vi "Configure Trigger (Runt).vi"(0 "VISA resource name":refnum<visa-resource-name>, 1 "Trigger Polarity (0: Positive)":u16(ring) items=["Positive", "Negative", "Either"], 5 "Trigger Source (0: Channel 1)":u16(ring) items=["Channel 1", "Channel 2", "Channel 3", "Channel 4", "RF"], 7 "High Threshold (0.8V)":dbl=0.8, 9 "Low Threshold (0.0V)":dbl, 11 "error in (no error)":errorcluster, 12 "Trigger Condition (0: Occurs)":u16(ring) items=["Occurs", "Less Than", "More Than", "Equal", "Not Equal"], 13 "Runt Width (4.0ns)":dbl=4e-09) -> (4 "VISA resource name out":refnum<visa-resource-name>, 15 "error out":errorcluster)   [LabVIEW 2013, in "Tektronix DPO MSO 2000 4000 Series.lvlib"]
doc: "Configures runt trigger settings for an oscilloscope. A runt trigger occurs when the trigger signal crosses one of the runt thresholds twice without crossing the other runt threshold."
uses:
  Tektronix DPO MSO 2000 4000 Series.lvlib
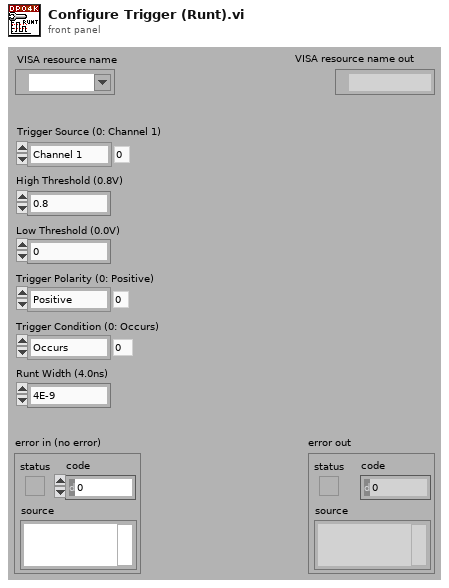
[diagram p1: front panel]
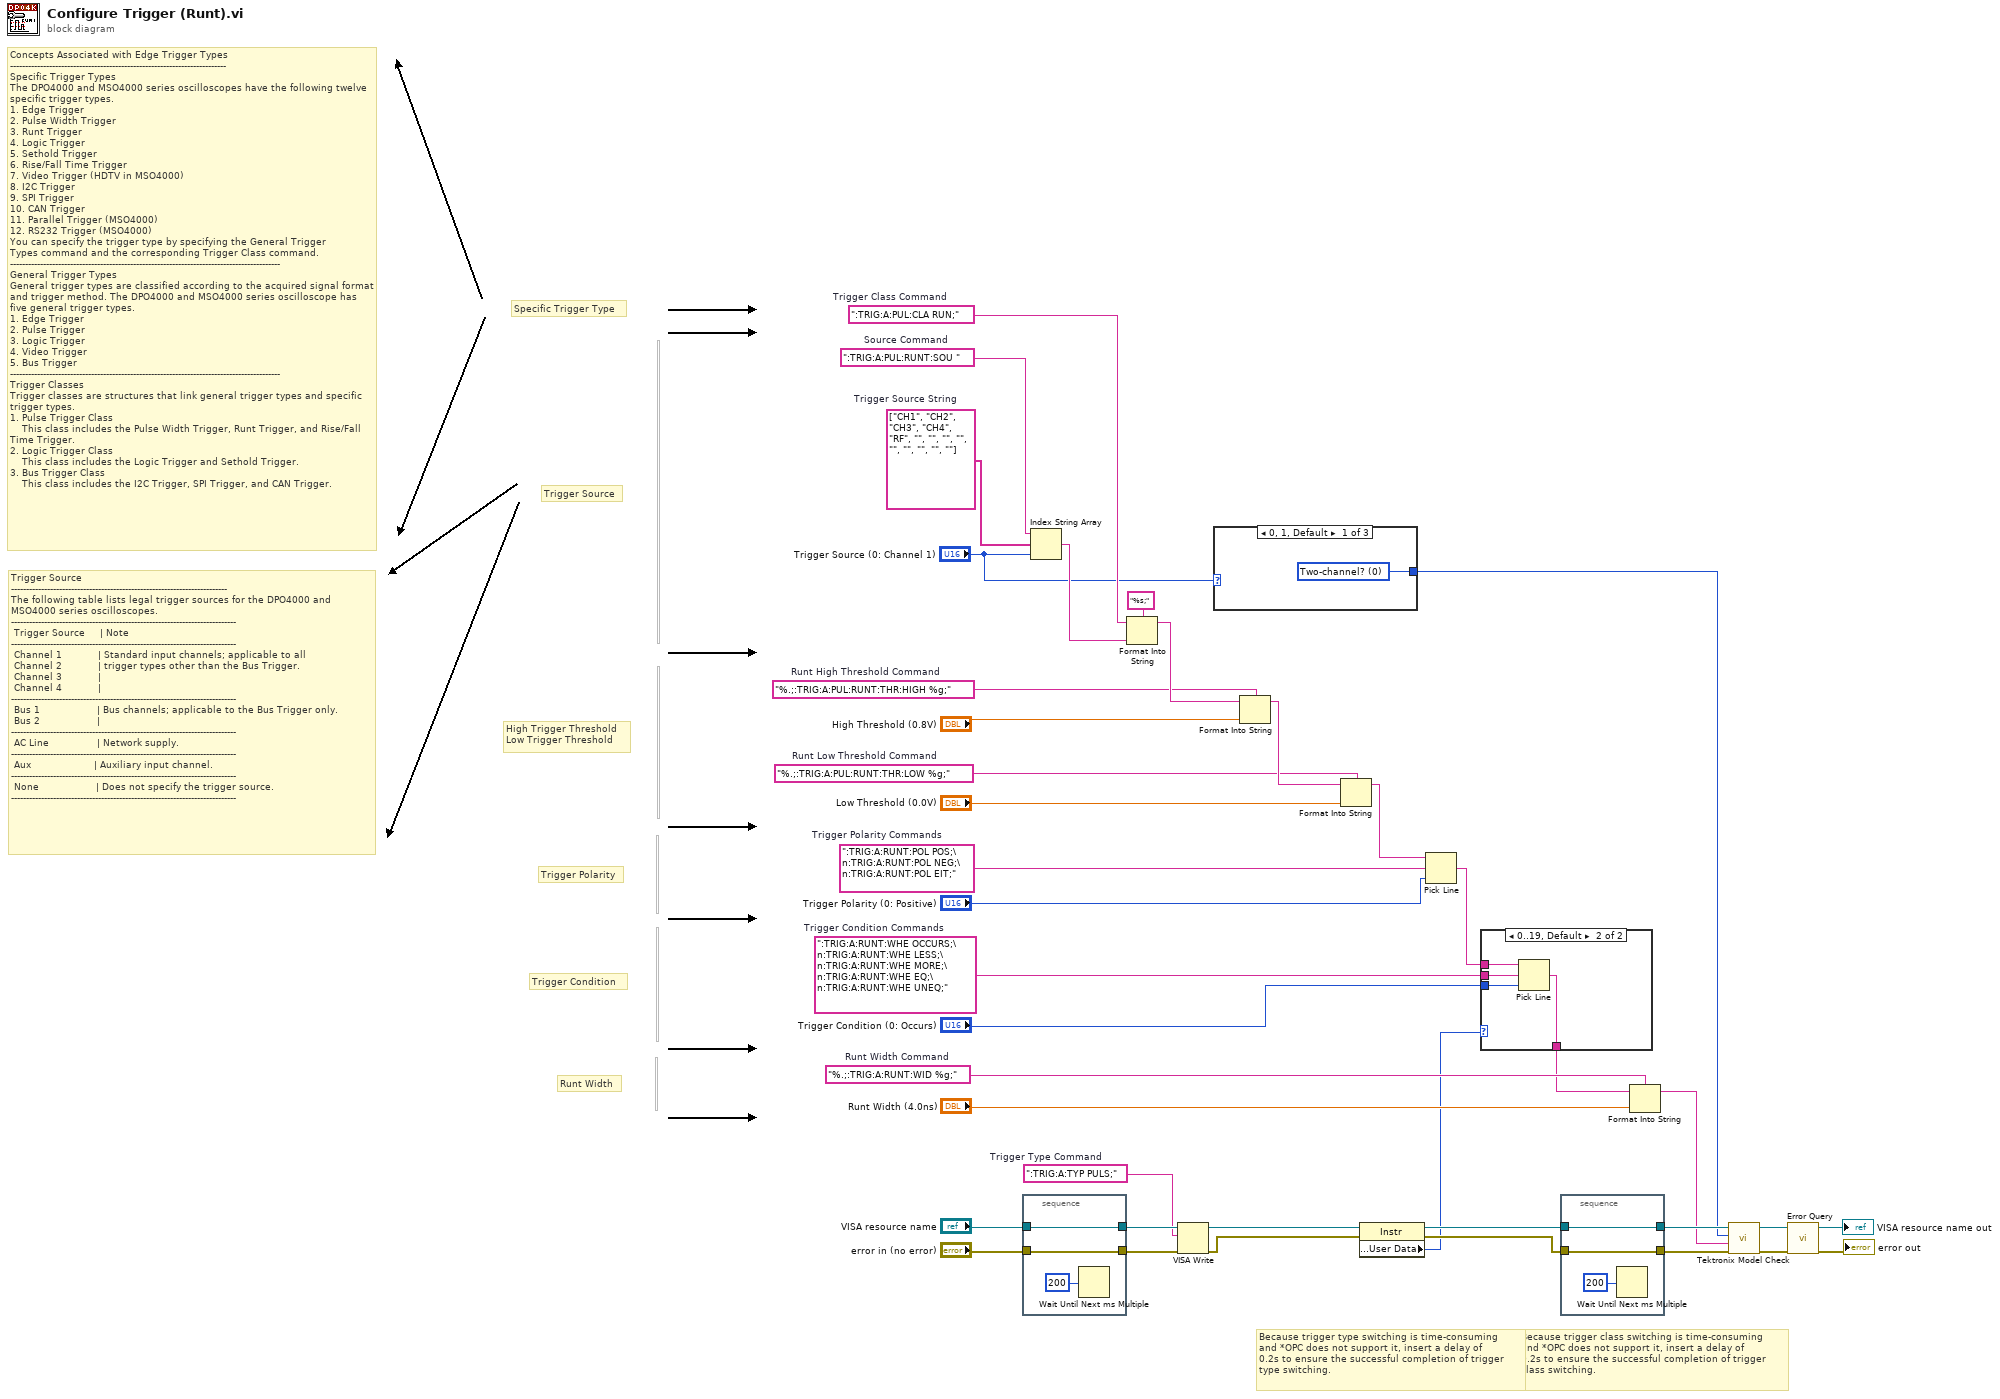
[diagram p0: block diagram]
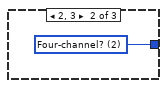
[diagram p2: hidden frame]
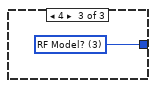
[diagram p3: hidden frame]
diagram:
  w17 = string[] ["CH1", "CH2", "CH3", "CH4", "RF", "", "", "", "", "", "", "", "", ""]  # Trigger Source String
  w21 = "%.;:TRIG:A:RUNT:WID %g;"  # Runt Width Command
  w24 = ":TRIG:A:RUNT:WHE OCCURS;\n:TRIG:A:RUNT:WHE LESS;\n:TRIG:A:RUNT:WHE MORE;\n:TRIG:A:RUNT:WHE EQ;\n:TRIG:A:RUNT:WHE UNEQ;"  # Trigger Condition Commands
  w26 = ":TRIG:A:RUNT:POL POS;\n:TRIG:A:RUNT:POL NEG;\n:TRIG:A:RUNT:POL EIT;"  # Trigger Polarity Commands
  w28 = "%.;:TRIG:A:PUL:RUNT:THR:LOW %g;"  # Runt Low Threshold Command
  w30 = "%.;:TRIG:A:PUL:RUNT:THR:HIGH %g;"  # Runt High Threshold Command
  w36 = ":TRIG:A:PUL:RUNT:SOU "  # Source Command
  w34 = ":TRIG:A:PUL:CLA RUN;"  # Trigger Class Command
  w37 = ":TRIG:A:TYP PULS;"  # Trigger Type Command
  # "Trigger Source\n------------------------------------------------------------------------\nThe following table lists legal trigger sources for the DPO4000 and MSO4000 series oscilloscopes.\n---------------------------------------------------------------------------\n Trigger Source     | Note                                                           \n---------------------------------------------------------------------------\n Channel 1            | Standard input channels; applicable to all      \n Channel 2            | trigger types other than the Bus Trigger.         \n Channel 3            |     \n Channel 4            |\n---------------------------------------------------------------------------\n Bus 1                   | Bus channels; applicable to the Bus Trigger only.\n Bus 2                   | \n---------------------------------------------------------------------------\n AC Line                | Network supply.\n---------------------------------------------------------------------------\n Aux                     | Auxiliary input channel.\n---------------------------------------------------------------------------\n None                   | Does not specify the trigger source.\n---------------------------------------------------------------------------"
  # "Concepts Associated with Edge Trigger Types\n------------------------------------------------------------------------\nSpecific Trigger Types\nThe DPO4000 and MSO4000 series oscilloscopes have the following twelve specific trigger types.\n1. Edge Trigger\n2. Pulse Width Trigger\n3. Runt Trigger\n4. Logic Trigger\n5. Sethold Trigger\n6. Rise/Fall Time Trigger\n7. Video Trigger (HDTV in MSO4000)\n8. I2C Trigger\n9. SPI Trigger\n10. CAN Trigger\n11. Parallel Trigger (MSO4000)\n12. RS232 Trigger (MSO4000)\nYou can specify the trigger type by specifying the General Trigger \nTypes command and the corresponding Trigger Class command.\n------------------------------------------------------------------------------------------\nGeneral Trigger Types \nGeneral trigger types are classified according to the acquired signal format and trigger method. The DPO4000 and MSO4000 series oscilloscope has five general trigger types.\n1. Edge Trigger\n2. Pulse Trigger\n3. Logic Trigger\n4. Video Trigger\n5. Bus Trigger\n------------------------------------------------------------------------------------------\nTrigger Classes\nTrigger classes are structures that link general trigger types and specific trigger types.\n1. Pulse Trigger Class\n    This class includes the Pulse Width Trigger, Runt Trigger, and Rise/Fall Time Trigger.\n2. Logic Trigger Class\n    This class includes the Logic Trigger and Sethold Trigger.\n3. Bus Trigger Class\n    This class includes the I2C Trigger, SPI Trigger, and CAN Trigger."
  # "Because trigger class switching is time-consuming\nand *OPC does not support it, insert a delay of\n0.2s to ensure the successful completion of trigger\nclass switching."
  # "Because trigger type switching is time-consuming\nand *OPC does not support it, insert a delay of\n0.2s to ensure the successful completion of trigger\ntype switching."
  # "Runt Width"
  # "Trigger Condition"
  # "Trigger Polarity"
  # "High Trigger Threshold\nLow Trigger Threshold"
  # "Trigger Source"
  # "Specific Trigger Type"
  n1 = stacked-sequence {
    tunnel: "VISA resource name" -> [w41]
    tunnel: [w41] -> w39
    tunnel: "error in (no error)" -> [w40]
    tunnel: [w40] -> w38
    frame #0 {
      n2 = Wait Until Next ms Multiple(millisecond multiple=u32 200) -> ()  [unwired: 1 out]
    }
  }
  n3 = Index String Array(1:"Trigger Source (0: Channel 1)", 2:w17, 3:w36) -> (0:w35:string)
  n4 = Format Into String(format string="%s;", initial string=w34, w35) -> (resulting string=w32:string)  [unwired: 1 in, 1 out]
  n5 = VISA Write(VISA resource name=w39, write buffer=w37, error in (no error)=w38) -> (VISA resource name out=w12:refnum<visa-resource-name>, error out=w11:errorcluster)  [unwired: 1 out]
  n6 = case shown="0, 1, Default" "Trigger Source (0: Channel 1)" {
    tunnel: [w43 w44 w45] -> w1
    frame 0, 1, Default {
      w43 = u16 0 items=["Two-channel?", "Digital Model?", "Four-channel?", "RF Model?"] ("Oscilloscope Model Tests (3: RF Model?)")
    }
    frame 2, 3 {
      w44 = u16 2 items=["Two-channel?", "Digital Model?", "Four-channel?", "RF Model?"] ("Oscilloscope Model Tests (3: RF Model?)")
    }
    frame 4 {
      w45 = u16 3 items=["Two-channel?", "Digital Model?", "Four-channel?", "RF Model?"] ("Oscilloscope Model Tests (3: RF Model?)")
    }
  }
  n7 = Format Into String(format string=w30, initial string=w32, "High Threshold (0.8V)") -> (resulting string=w29:string)  [unwired: 1 in, 1 out]
  n8 = Format Into String(format string=w28, initial string=w29, "Low Threshold (0.0V)") -> (resulting string=w16:string)  [unwired: 1 in, 1 out]
  n9 = property class="Instr"(reference=w12, error in=w11) -> (reference out=w10:refnum<visa-resource-name>, error out=w9:errorcluster, "General Settings:User Data"=w8:u32)
  n10 = Pick Line(string ("")=w16, multi-line string=w26, line index="Trigger Polarity (0: Positive)") -> (output string=w15:string)
  n11 = case shown="0..19, Default" w8 {
    tunnel: w24 -> [_ w50]
    tunnel: "Trigger Condition (0: Occurs)" -> [_ w49]
    tunnel: [w46 w48] -> w20
    tunnel: w15 -> [w46 w47]
    frame 20, 27 {
    }
    frame 0..19, Default {
      n12 = Pick Line(string ("")=w47, multi-line string=w50, line index=w49) -> (output string=w48:string)
    }
  }
  n13 = stacked-sequence {
    tunnel: w10 -> [w52]
    tunnel: [w52] -> w7
    tunnel: w9 -> [w51]
    tunnel: [w51] -> w6
    frame #0 {
      n14 = Wait Until Next ms Multiple(millisecond multiple=u32 200) -> ()  [unwired: 1 out]
    }
  }
  n15 = Format Into String(format string=w21, initial string=w20, "Runt Width (4.0ns)") -> (resulting string=w3:string)  [unwired: 1 in, 1 out]
  n16 = call "Tektronix Model Check.vi"("error in (no error)"=w6, "Command String"=w3, "Oscilloscope Model Tests (3: RF Model?)"=w1, "VISA resource name"=w7) -> ("error out"=w4:errorcluster, "VISA resource name out"=w5:refnum<visa-resource-name>)  [unwired: 6 in]
  n17 = call "Error Query.vi"("error in (no error)"=w4, "VISA resource name"=w5) -> ("error out"=→"error out":errorcluster, "VISA resource name out"=→"VISA resource name out":refnum<visa-resource-name>)  [unwired: 6 in, 2 out]
